vi "Parse Profile Step.vi"(0 "CmdCluster In":T1, 7 "StepColumn":string[](array[string]), 11 "Brushed?":bool) -> (4 "CmdCluster Out":T1)   [LabVIEW 2013]
uses:
  TypeDef/Command Cluster.ctl
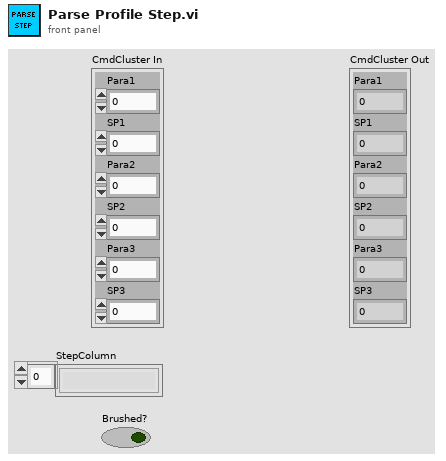
[diagram p1: front panel]
types:
  T1 = typedef "Command Cluster.ctl" = cluster{"Para1":i32, "SP1":dbl, "Para2":i32, "SP2":dbl, "Para3":i32, "SP3":dbl}
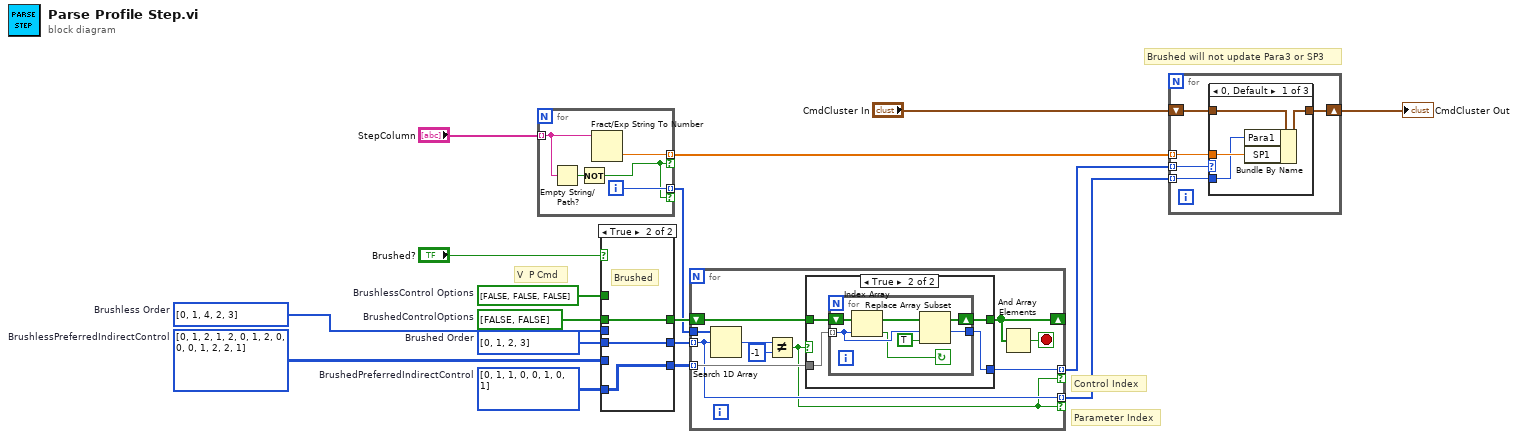
[diagram p0: block diagram]
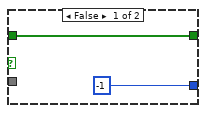
[diagram p2: hidden frame]
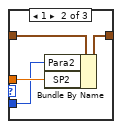
[diagram p3: hidden frame]
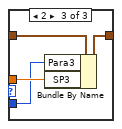
[diagram p4: hidden frame]
diagram:
  w16 = i32[] [0, 1, 2, 3]  # Brushed Order
  w17 = i32[] [0, 1, 4, 2, 3]  # Brushless Order
  w14 = bool[] [FALSE, FALSE, FALSE]  # BrushlessControl Options
  w15 = i32[][] [[0, 1, 2, 1, 2], [0, 1, 2, 0, 0], [0, 1, 2, 2, 1]]  # BrushlessPreferredIndirectControl
  w13 = bool[] [FALSE, FALSE]  # BrushedControlOptions
  w12 = i32[][] [[0, 1, 1, 0], [0, 1, 0, 1]]  # BrushedPreferredIndirectControl
  # "Brushed will not update Para3 or SP3"
  # "Parameter Index"
  # "Control Index"
  # "V  P Cmd"
  n1 = for {
    tunnel: "StepColumn" -> [w19] mode=indexing
    tunnel: [w22] -> w5 mode=indexing if=w18
    tunnel: [w21] -> w8 mode=indexing if=w18
    i -> [w21]
    n2 = Empty String/Path?(string/path=w19) -> (empty?=w20:bool)
    n3 = Not(x=w20) -> (.not. x?=w18:bool)
    n4 = Fract/Exp String To Number(string=w19) -> (number=w22:dbl)  [unwired: 3 in, 1 out]
  }
  n5 = case shown="True" "Brushed?" {
    tunnel: w12 -> [_ w27]
    tunnel: w13 -> [_ w28]
    tunnel: w14 -> [w25 _]
    tunnel: w15 -> [w23 _]
    tunnel: w16 -> [_ w26]
    tunnel: w17 -> [w24 _]
    tunnel: [w25 w28] -> w9
    tunnel: [w24 w26] -> w7
    tunnel: [w23 w27] -> w6
    frame False {
      # "Brushless"
    }
    frame True {
      # "Brushed"
    }
  }
  n6 = for {
    tunnel: w6 -> [w32] mode=indexing
    shift-right: [w34] -> _
    shift-left: w9 -> [w33]
    tunnel: w8 -> [w38]
    tunnel: w7 -> [w30] mode=indexing
    tunnel: [w31] -> w4 mode=indexing if=w29
    tunnel: [w30] -> w3 mode=indexing if=w29
    stop <- w35 stop-if-true
    n7 = Search 1D Array(1D array=w38, element=w30) -> (index of element=w37:i32)  [unwired: 1 in]
    n8 = Not Equal?(x=w37, y=-1) -> (x != y?=w29:bool)
    n9 = case shown="True" w29 {
      tunnel: [w40 w42] -> w34
      tunnel: w33 -> [w40 w42]
      tunnel: w32 -> [_ w43]
      tunnel: [-1 w41] -> w31
      frame False {
      }
      frame True {
        n10 = for {
          shift-right: [w47] -> _
          shift-left: w42 -> [w48]
          tunnel: w43 -> [w45] mode=indexing
          tunnel: [w45] -> w41
          stop <- w44 continue-if-true
          n11 = Index Array(array=w48, index=w45) -> (element=w44:bool)
          n12 = Replace Array Subset(array=w48, new element=TRUE ("new element/subarray"), index=w45) -> (w47:bool[])
        }
      }
    }
    n13 = And Array Elements(Boolean array=w34) -> (logical AND=w35:bool)
  }
  n14 = for {
    tunnel: w5 -> [w50] mode=indexing
    tunnel: w4 -> [w53] mode=indexing
    shift-right: [w51] -> w1
    shift-left: "CmdCluster In" -> [w52]
    tunnel: w3 -> [w49] mode=indexing
    n15 = case shown="0, Default" w53 {
      tunnel: w52 -> [w57 w61 w65]
      tunnel: [w56 w60 w64] -> w51
      tunnel: w50 -> [w55 w59 w63]
      tunnel: w49 -> [w54 w58 w62]
      frame 0, Default {
        n16 = Bundle By Name(cluster=w57, "Para1"=w54, "SP1"=w55) -> (w56:T1)
      }
      frame 1 {
        n17 = Bundle By Name(cluster=w61, "Para2"=w58, "SP2"=w59) -> (w60:T1)
      }
      frame 2 {
        n18 = Bundle By Name(cluster=w65, "Para3"=w62, "SP3"=w63) -> (w64:T1)
      }
    }
  }
  "CmdCluster Out" <- w1
